vi "oax_Build Digital Tacho and Vibration Output Signal.vi"(7 "reset? (T)":bool=TRUE, 8 "error in (no error)":errorcluster, 11 "input cluster":T2) -> (0 "error out":errorcluster, 2 "waveform data":waveform(dbl)[](array[waveform]), 3 "digital tacho info":T1)   [LabVIEW 2017]
uses:
  <vilib>/addons/Sound and Vibration/Order Analysis/Tach Process/SubVIs/digital tach info.ctl
  <vilib>/Waveform/WDTOps.llb/WDT Append Waveforms DBL.vi
  <vilib>/addons/Sound and Vibration/Order Analysis/Tach Process/SoundVib_TachProcess.lvlib
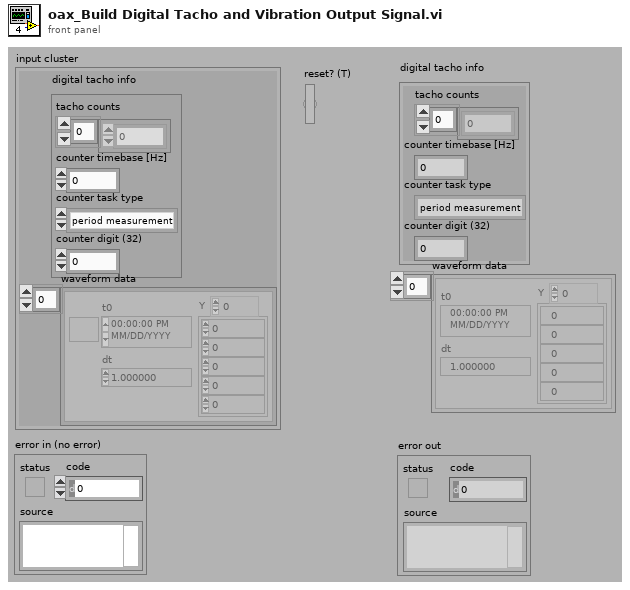
[diagram p1: front panel]
types:
  T1 = typedef "SoundVib_TachProcess.lvlib/digital tach info.ctl" = cluster{"tacho counts":i64[], "counter timebase [Hz]":dbl, "counter task type":enum16{"period measurement", "event counting"}, "counter digit (32)":i32}
  T2 = cluster{"digital tacho info":T1, "waveform data":waveform(dbl)[]}
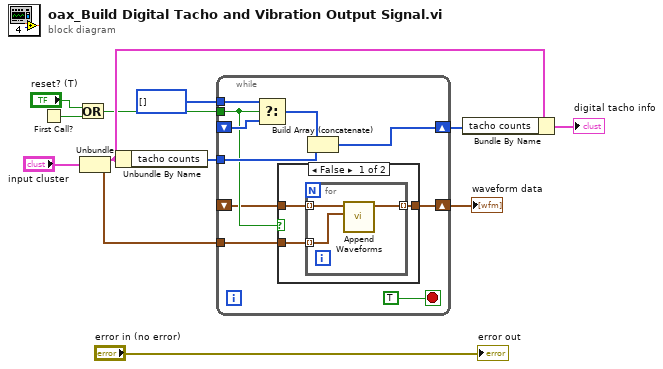
[diagram p0: block diagram]
diagram:
  n1 = First Call?() -> (First Call?: T/F=w3:bool)
  n2 = Or(x="reset? (T)", y=w3) -> (x .or. y?=w2:bool)
  n3 = Unbundle("input cluster") -> ("digital tacho info"=w7:T1, "waveform data"=w10:waveform(dbl)[])
  n4 = Unbundle By Name(w7) -> ("tacho counts"=w8:i64[])
  n5 = while {
    tunnel: w8 -> [w16]
    shift-right: [w22] -> w6
    shift-left: _ -> [w21]
    tunnel: w2 -> [w14]
    tunnel: u32[] [] ("t") -> [w20]
    tunnel: w10 -> [w18]
    shift-right: [w17] -> w9
    shift-left: _ -> [w13]
    stop <- TRUE stop-if-true
    n6 = Select(t=w20, s=w14, f=w21) -> (s? t:f=w19:i64[])
    n7 = case shown="False" w14 {
      tunnel: w18 -> [w25 w29]
      tunnel: [w24 w29] -> w17
      tunnel: w13 -> [w23 _]
      frame False {
        n8 = for {
          tunnel: w25 -> [w28] mode=indexing
          tunnel: [w27] -> w24 mode=indexing
          tunnel: w23 -> [w26] mode=indexing
          n9 = call-poly <vilib>:"Append Waveforms.vi"("waveform B"=w28, "waveform A"=w26) -> ("waveform out"=w27:waveform(dbl))  [unwired: 8 in, 1 out]
        }
      }
      frame True {
      }
    }
    n10 = Build Array (concatenate)(w19, w16) -> (w22:i64[])
  }
  "waveform data" <- w9
  n11 = Bundle By Name(cluster=w7, "tacho counts"=w6) -> (→"digital tacho info":T1)
  "error out" <- "error in (no error)"
